vi "Set Channel Current.vi"(8 "error in (no error)":errorcluster, 9 "Channel Select":enum16{"Channel 1", "Channel 2", "Channel 3"}(ring), 10 "Current":dbl format="%#_13g", 11 "2230G in":refnum<class "2230G.lvclass">) -> (0 "error out":errorcluster, 3 "2230G out":refnum<class "2230G.lvclass">)   [LabVIEW 2018, in "2230G.lvlib" / "2230G.lvclass"]
uses:
  2230G.lvclass
  2230G.lvclass/2230G.ctl
  PPLs/Power Supply/Parent/Power_Supply.lvlibp/Power Supply.lvclass
  <instrlib>/Keithley KE22xx Series/Keithley KE22xx Series.lvlib
  C:/Projects/LabVIEW/PPLs/Power Supply/Parent/Power_Supply.lvlibp/Power Supply.lvclass
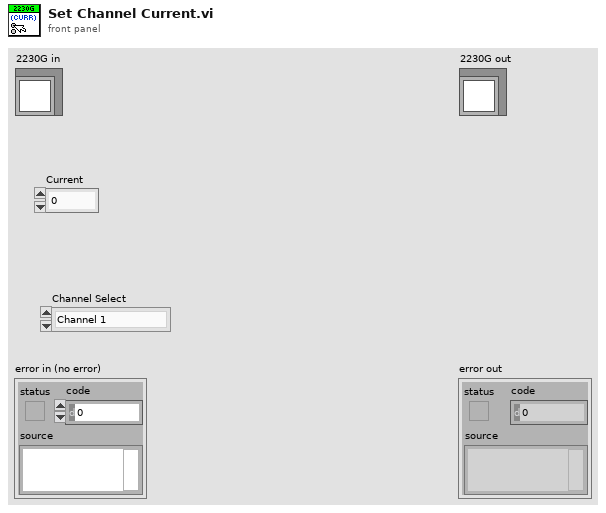
[diagram p1: front panel]
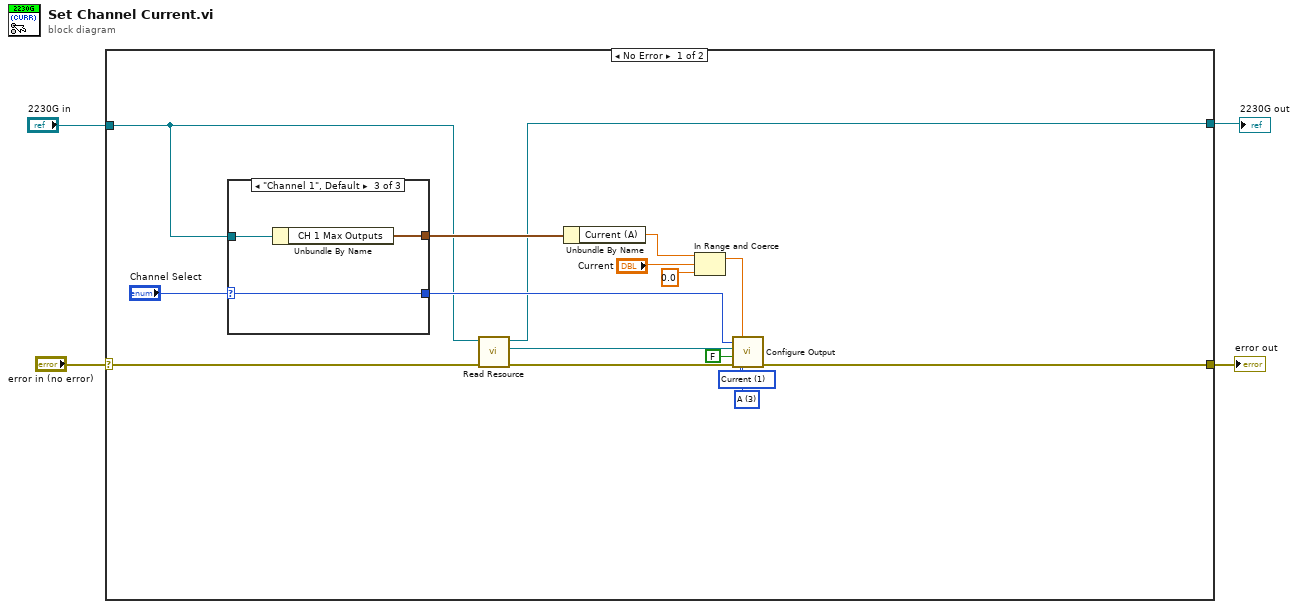
[diagram p0: block diagram]
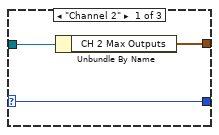
[diagram p2: hidden frame]
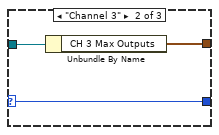
[diagram p3: hidden frame]
diagram:
  n1 = case shown="No Error" "error in (no error)" {
    selector: "error in (no error)" -> [w9 w31]
    tunnel: [w6 w31] -> w1
    tunnel: [w7 w30] -> w3
    tunnel: "2230G in" -> [w10 w30]
    frame No Error {
      w5 = u16 3 items=["V", "mV", "kV", "A", "mA"] ("Unit(V)")
      w15 = u16 1 items=["Voltage", "Current"] ("Function(0:Voltage)")
      n2 = case shown="\"Channel 1\", Default" "Channel Select" {
        selector: "Channel Select" -> [w21 w24 w27]
        tunnel: w10 -> [w23 w25 w29]
        tunnel: [w22 w26 w28] -> w19
        tunnel: [w21 w24 w27] -> w11
        frame "Channel 2" {
          n3 = Unbundle By Name(w23) -> ("CH 2 Max Outputs"=w22:cluster{"Voltage (V)":dbl, "Current (A)":dbl})
        }
        frame "Channel 3" {
          n4 = Unbundle By Name(w25) -> ("CH 3 Max Outputs"=w26:cluster{"Voltage (V)":dbl, "Current (A)":dbl})
        }
        frame "Channel 1", Default {
          n5 = Unbundle By Name(w29) -> ("CH 1 Max Outputs"=w28:cluster{"Voltage (V)":dbl, "Current (A)":dbl})
        }
      }
      n6 = call "Read Resource.vi"("error in"=w9, "Power Supply in"=w10) -> ("error out"=w12:errorcluster, "Resource"=w13:refnum<visa-resource-name>, "Power Supply out"=w7:refnum<class "2230G.lvclass">)  [unwired: 7 in]
      n7 = Unbundle By Name(w19) -> ("Current (A)"=w18:dbl)
      n8 = In Range and Coerce(upper limit=w18, x="Current", lower limit=0.0) -> (coerced(x)=w8:dbl)  [unwired: 1 out]
      n9 = call <instrlib>:"Configure Output.vi"("VISA resource name"=w13, "Manual Range(0.00)"=w8, "Channel Select"=w11, "Function(0:Voltage)"=w15, "Enable Output (T: Enable)"=FALSE, "error in (no error)"=w12, "Unit(V)"=w5) -> ("error out"=w6:errorcluster)  [unwired: 7 in, 1 out]
    }
    frame Error {
    }
  }
  "error out" <- w1
  "2230G out" <- w3
